vi "SyringeTool Class Sandbox.vi"() -> ()   [LabVIEW 2011]
uses:
  SyringeTool Class.lvclass
panel:
  out "error out":errorcluster
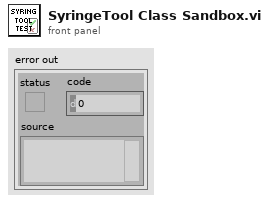
[diagram p1: front panel]
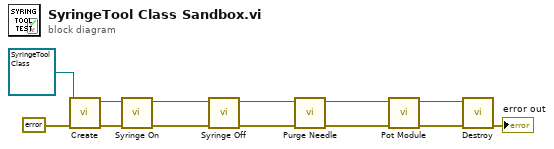
[diagram p0: block diagram]
diagram:
  n1 = call-dynamic "Create.vi"("error in (no error)"=errorcluster {"status"=FALSE, "code"=0, "source"=""} ("error constant"), "SyringeTool Class in"=refnum<class "SyringeTool Class.lvclass"> refnum) -> ("error out"=w8:errorcluster, "SyringeTool Class out"=w13:refnum<class "SyringeTool Class.lvclass">)  [unwired: 8 in]
  n2 = call "Syringe On.vi"("error in (no error)"=w8, "SyringeTool Class in"=w13) -> ("error out"=w7:errorcluster, "SyringeTool Class out"=w12:refnum<class "SyringeTool Class.lvclass">)  [unwired: 8 in]
  n3 = call "Syringe Off.vi"("error in (no error)"=w7, "SyringeTool Class in"=w12) -> ("error out"=w6:errorcluster, "SyringeTool Class out"=w11:refnum<class "SyringeTool Class.lvclass">)  [unwired: 8 in]
  n4 = call "Purge Needle.vi"("error in (no error)"=w6, "SyringeTool Class in"=w11) -> ("error out"=w5:errorcluster, "SyringeTool Class out"=w10:refnum<class "SyringeTool Class.lvclass">)  [unwired: 8 in]
  n5 = call "Pot Module.vi"("error in (no error)"=w5, "SyringeTool Class in"=w10) -> ("error out"=w4:errorcluster, "SyringeTool Class out"=w9:refnum<class "SyringeTool Class.lvclass">)  [unwired: 8 in]
  n6 = call-dynamic "Destroy.vi"("error in (no error)"=w4, "SyringeTool Class in"=w9) -> ("error out"=→"error out":errorcluster)  [unwired: 8 in, 1 out]
